vi "TestExec.Status, String to PASS.vi"(11 "String":string) -> (3 "PASS":bool)   [LabVIEW 2019]
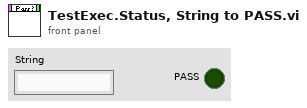
[diagram p1: front panel]
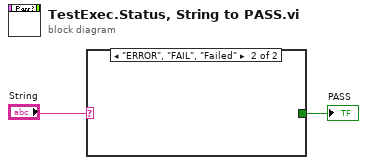
[diagram p0: block diagram]
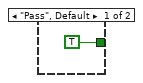
[diagram p2: hidden frame]
diagram:
  n1 = case shown="\"ERROR\", \"FAIL\", \"Failed\"" "String" {
    tunnel: [TRUE _] -> w1
    frame "Pass", Default {
    }
    frame "ERROR", "FAIL", "Failed" {
    }
  }
  "PASS" <- w1
